vi "sendSetServoDefaultPosition.vi"(1 "servo position":u16(knob)=260 min=260 max=1150 step=1 scale=260.0..1150.0, 2 "channel":u8 max=15 step=1) -> ()   [LabVIEW 2011]
uses:
  GlobalSerial.vi
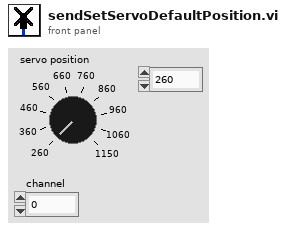
[diagram p1: front panel]
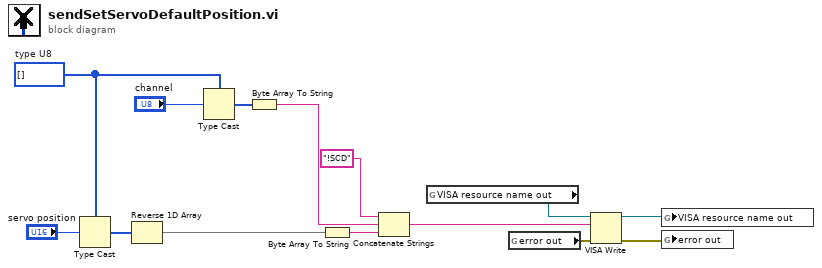
[diagram p0: block diagram]
diagram:
  w8 = u8[] []  # type U8
  n1 = Type Cast(type=w8, x="servo position") -> (*(type *) &x=w12:u8[])
  n2 = Reverse 1D Array(array=w12) -> (reversed array=w7:u8[])
  n3 = Type Cast(type=w8, x="channel") -> (*(type *) &x=w10:u8[])
  n4 = Byte Array To String(unsigned byte array=w10) -> (string=w11:string)
  n5 = Byte Array To String(unsigned byte array=w7) -> (string=w1:string)
  n6 = Concatenate Strings("!SCD" ("string"), w11, w1) -> (w6:string)
  n7 = global read "GlobalSerial.vi" "VISA resource name out"() -> (w3:refnum<visa-resource-name>)
  n8 = global read "GlobalSerial.vi" "error out"() -> (w5:errorcluster)
  n9 = VISA Write(VISA resource name=w3, write buffer=w6, error in (no error)=w5) -> (VISA resource name out=w2:refnum<visa-resource-name>, error out=w4:errorcluster)  [unwired: 1 out]
  n10 = global write "GlobalSerial.vi" "VISA resource name out"(w2) -> ()
  n11 = global write "GlobalSerial.vi" "error out"(w4) -> ()
